vi "test_Set Pattern.vi"(8 "error in (no error)":errorcluster, 11 "IO Lines Patttern Settings":T1[](array[typedef]) {"Duration (us)" min=0.005 max=42550000.0 step=0.005 format="%#.3f"}) -> (0 "error out":errorcluster, 2 "Pattern Digital Data":digitaldata, 3 "Data out":u64[](array[numeric])=[5631702913073631, 5629503829180420, 5629508124147720, 5629503829180426, 5629508124147722, 5629503829180426, 5629508124147722, 5629503829180426, 5629508124147722, 5631707147403291])   [LabVIEW 2016]
uses:
  Host/Typedefs/IO Lines State.ctl
  Host/Typedefs/LV2G Operation.ctl
  Host/Typedefs/IO Buffer Operation.ctl
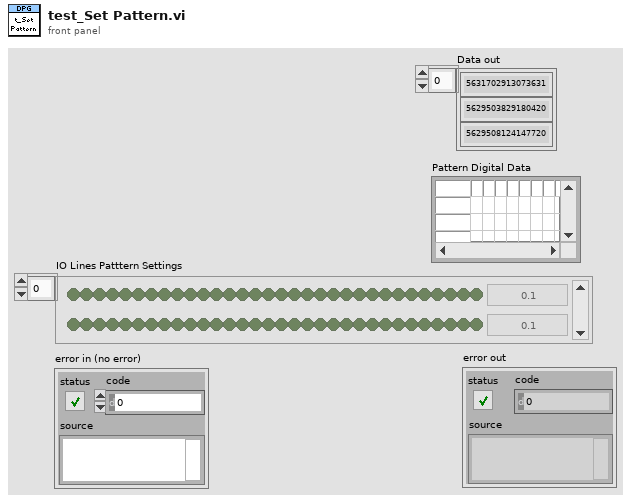
[diagram p1: front panel]
types:
  T1 = typedef "IO Lines State.ctl" = cluster{"State":bool[], "Duration (us)":dbl}
  T2 = typedef "IO Buffer Operation.ctl" = enum16{"Initialize", "Write IO Data_Rd", "Read IO Data_Rd", "Write IO Data_Wr", "Read IO Data_Wr", "Write  IO Data_Dir", "Read  IO Data_Dir", "Write Host to Target FIFO", "Read Host to Target FIFO", "Write Target to Host FIFO", "Read Target to Host FIFO", "Write Monitor Enable?", "Read Monitor Enable?", "Close"}
  T3 = typedef "LV2G Operation.ctl" = enum16{"Initialize", "Set", "Get", "Close"}
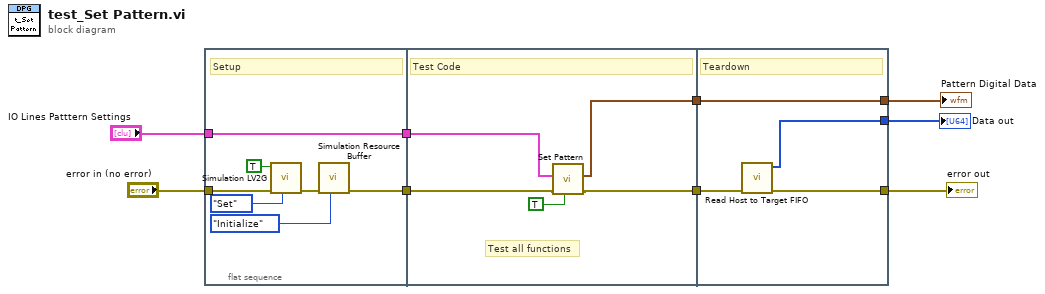
[diagram p0: block diagram]
diagram:
  n1 = flat-sequence {
    tunnel: "error in (no error)" -> [w16]
    tunnel: [w11] -> w9
    tunnel: [w10] -> w4
    tunnel: "IO Lines Patttern Settings" -> [w10]
    tunnel: w9 -> [w21]
    tunnel: [w20] -> w8
    tunnel: w4 -> [w18]
    tunnel: [w17] -> w2
    tunnel: [w24] -> w6
    tunnel: w8 -> [w25]
    tunnel: [w23] -> w5
    tunnel: w2 -> [w22]
    tunnel: [w22] -> w1
    frame #0 {
      # "Setup"
      n2 = call "Simulation LV2G.vi"("Operation (Get)"=LV2G_Operation."Set", "error in (no error)"=w16, "Simulation?"=TRUE) -> ("error out"=w13:errorcluster)  [unwired: 7 in, 1 out]
      n3 = call "Simulation Resource Buffer.vi"("IO Buffer Operation"=IO_Buffer_Operation."Initialize", "error in (no error)"=w13) -> ("error out"=w11:errorcluster)  [unwired: 7 in, 2 out]
    }
    frame #1 {
      # "Test all functions"
      # "Test Code"
      n4 = call "Set Pattern.vi"("Write to FPGA(T)"=TRUE, "error in (no error)"=w21, "IO Lines Patttern Settings"=w18) -> ("error out"=w20:errorcluster, "Pattern Digital Data"=w17:digitaldata)  [unwired: 5 in, 1 out]
    }
    frame #2 {
      # "Teardown"
      n5 = call "Read Host to Target FIFO.vi"("error in (no error)"=w25) -> ("error out"=w24:errorcluster, "Host to Target FIFO"=w23:u64[])  [unwired: 9 in]
    }
  }
  "error out" <- w6
  "Data out" <- w5
  "Pattern Digital Data" <- w1
